vi "Get Status.vi"(8 "error in (no error)":errorcluster) -> (0 "error out":errorcluster, 2 "No. Of Elements in Queue":i32, 3 "Queue Name":string)   [LabVIEW 2022 SP3]
doc: "Returns the queue name and number of elements currently in the queue. Does not remove (dequeue) any element from the queue."
panel:
  # "Development\ncontrols/indicators useful for development and testing, but which are not outputs of the VI"
  # "Input\nInputs to the VI"
  # "Output\nOutputs of the VI"
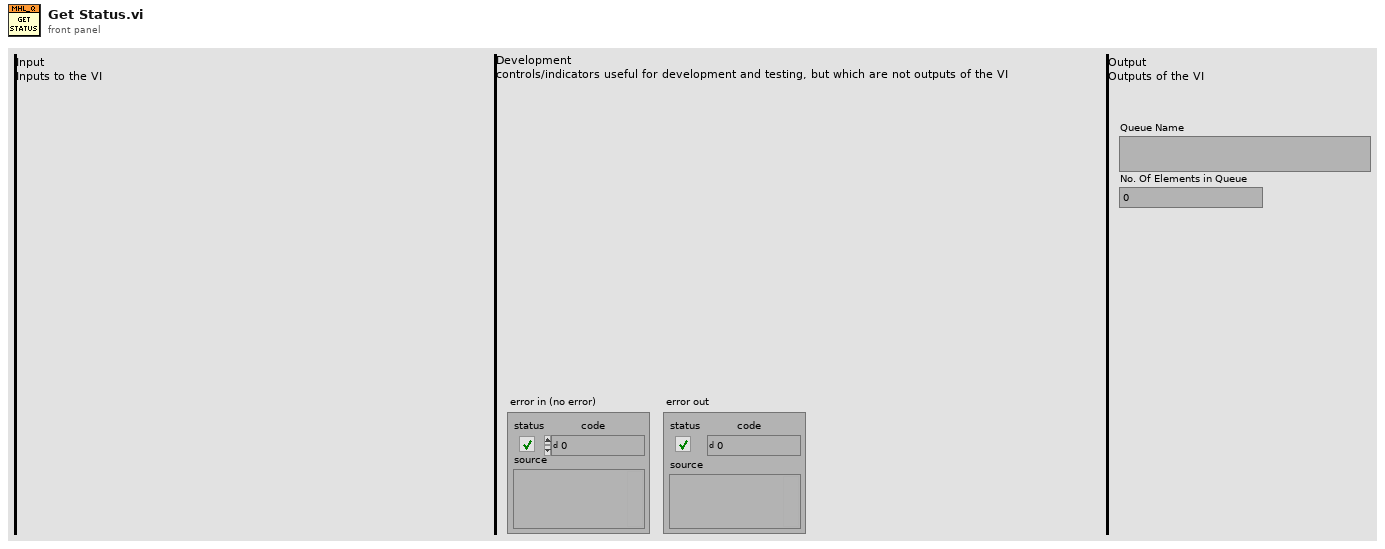
[diagram p1: front panel]
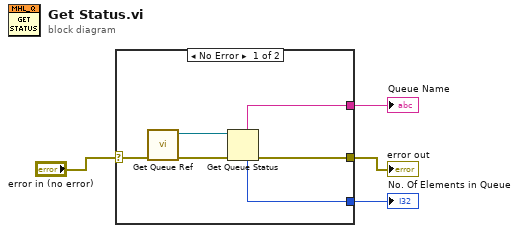
[diagram p0: block diagram]
diagram:
  n1 = case shown="No Error" "error in (no error)" {
    selector: "error in (no error)" -> [w10 w11]
    tunnel: [w9 w11] -> w3
    tunnel: [w6 _] -> w2
    tunnel: [w5 _] -> w1
    frame No Error {
      n2 = call "Get Queue Ref.vi"("error in (no error)"=w10) -> ("error out"=w7:errorcluster, "Queue Ref"=w8:refnum<queue>)  [unwired: 9 in]
      n3 = Get Queue Status(queue=w8, error in (no error)=w7) -> (queue name=w5:string, error out=w9:errorcluster, # elements in queue=w6:i32)  [unwired: 1 in, 5 out]
    }
    frame Error {
    }
  }
  "error out" <- w3
  "No. Of Elements in Queue" <- w2
  "Queue Name" <- w1
